vi "ConfigMessageMetadata.vi"(7 "Message":refnum<class "Message.lvclass">, 9 "TellOrigin":T1, 10 "Lifetime":T2, 11 "ActorAlias":string) -> (5 "Message":refnum<class "Message.lvclass">)   [LabVIEW 2020, in "jettl.lvlib" / "Message.lvclass"]
uses:
  Message.lvclass
  Lifecycle.ctl
  jettl.lvlib
  TellOrigin.ctl
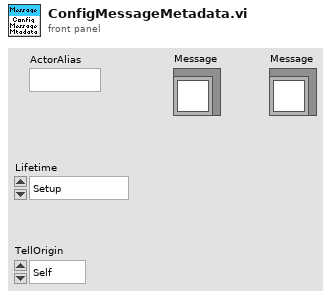
[diagram p1: front panel]
types:
  T1 = typedef "jettl.lvlib/TellOrigin.ctl" = enum16{"Self", "Mediator", "Component"}
  T2 = typedef "jettl.lvlib/Lifecycle.ctl" = enum16{"Setup", "TeardownBeforeStart", "Start", "Running", "Stop", "TeardownAfterStart"}
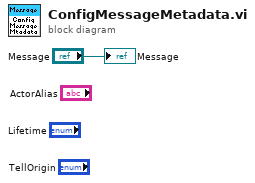
[diagram p0: block diagram]
diagram:
  "Message" <- "Message"
